vi "RunMe (Test Launcher).vi"() -> ()   [LabVIEW 2023, in "caraya unit tests.lvclass"]
uses:
  caraya unit tests.lvclass
  <vilib>/addons/_JKI Toolkits/Caraya/classes/Test Runner/Test Runner.lvclass
panel:
  out "error out":errorcluster
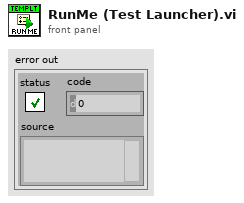
[diagram p1: front panel]
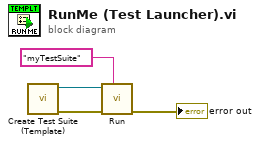
[diagram p0: block diagram]
diagram:
  n1 = call "Create Test Suite (Template).vi"() -> ("error out"=w3:errorcluster, "Test Runner.Template out"=w4:refnum<class "caraya unit tests.lvclass">)  [unwired: 10 in]
  n2 = call <vilib>:"Run.vi"("Name"="myTestSuite", "error in (no error)"=w3, "Test Runner in"=w4) -> ("error out"=→"error out":errorcluster)  [unwired: 6 in, 2 out]
